vi "Verify with 3 Scrubbers.vi"(8 "error in":errorcluster) -> (0 "error out":errorcluster)   [LabVIEW 2020, in "Scrubber.Tests.lvclass"]
uses:
  Scrubber.Tests.lvclass
  Source/Approval Tests/Options/Options.lvclass
  Source/Approval Tests/Regex Scrubber/Regex Scrubber.lvclass
  C:/Users/SAS/Desktop/ApprovalTests.LabVIEW/Source/Approval Tests/Scrubber/Scrubber.lvclass
  Source/Approval Tests/Regex Scrubber/Regex Scrubber.lvclass/Regex Scrubber.ctl
  Source/Approval Tests/Options/Options.lvclass/Options.ctl
  Source/Approval Tests/Naming Data/Naming Data.lvclass/Naming Data.ctl
  4b862e9e-fcb2-487f-ab73-d9f83fbf4d2c.vi
  Source/Approval Tests/Regex Scrubber/Write Regex.vi
  Source/Approval Tests/Regex Scrubber/Write Replacement.vi
  4b862e9e-fcb2-487f-ab73-d9f83fbf4d2c.vi/500b534b-d6f0-4fa5-90b2-c40158375321.vi
  Source/Approval Tests/Update Test Name if Not Defined.vi
  4b862e9e-fcb2-487f-ab73-d9f83fbf4d2c.vi/500b534b-d6f0-4fa5-90b2-c40158375321.vi/93c5622b-9fb7-41e0-8c76-3fde37e94e34.vi
  Source/Approval Tests/Verify Core.vi
  Source/Approval Tests/Options/Read Scrubber.vi
  Source/Approval Tests/Naming Data/Read Test VI Name.vi
  Source/Approval Tests/Naming Data/Write Test VI Name.vi
  4b862e9e-fcb2-487f-ab73-d9f83fbf4d2c.vi/500b534b-d6f0-4fa5-90b2-c40158375321.vi/93c5622b-9fb7-41e0-8c76-3fde37e94e34.vi/04cb982b-2eda-40d0-8d7e-90f8e0b569b2.vi
  Source/Approval Tests/Options/Read Namer.vi
  Source/Approval Tests/Options/Read Naming Data.vi
  Source/Approval Tests/Options/Read Reporter.vi
  Source/Approval Tests/Options/Write Add Scrubber.vi
  Source/Approval Tests/conv EOL.vi
  <vilib>/Utility/libraryn.llb/Check if File or Folder Exists.vi
  Source/Approval Tests/Reporter/Report.vi
  <vilib>/addons/_JKI Toolkits/Caraya/classes/Assert/Assert.vi
  <vilib>/addons/_JKI Toolkits/Caraya/classes/Assert/Assert True.vi
  Source/Approval Tests/Scrubber/Scrubber.lvclass
  Source/Approval Tests/Namer/Namer.lvclass
  Source/Approval Tests/Naming Data/Naming Data.lvclass
  Source/Approval Tests/Reporter/Reporter.lvclass
  Scrubber.Tests.lvclass/Scrubber.Tests.ctl
  <vilib>/addons/_JKI Toolkits/Caraya/classes/Test/Test.lvclass
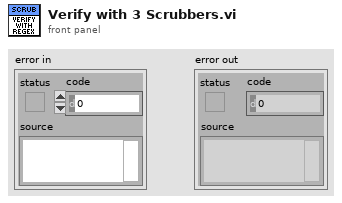
[diagram p1: front panel]
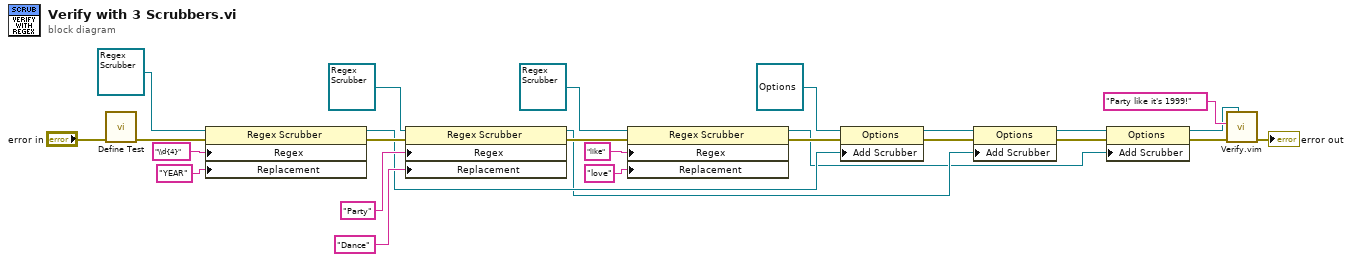
[diagram p0: block diagram]
diagram:
  n1 = call <vilib>:"Define Test.vi"("error in (no error)"="error in") -> ("error out"=w26:errorcluster)  [unwired: 9 in, 1 out]
  n2 = property class="Regex Scrubber"(reference=refnum<class "Regex Scrubber.lvclass"> refnum ("Approval Tests.lvlib:Regex Scrubber.lvclass"), error in=w26, "Regex"="\\d{4}", "Replacement"="YEAR") -> (reference out=w9:refnum<class "Regex Scrubber.lvclass">, error out=w23:errorcluster)
  n3 = property class="Regex Scrubber"(reference=refnum<class "Regex Scrubber.lvclass"> refnum ("Approval Tests.lvlib:Regex Scrubber.lvclass"), error in=w23, "Regex"="Party", "Replacement"="Dance") -> (reference out=w7:refnum<class "Regex Scrubber.lvclass">, error out=w22:errorcluster)
  n4 = property class="Regex Scrubber"(reference=refnum<class "Regex Scrubber.lvclass"> refnum ("Approval Tests.lvlib:Regex Scrubber.lvclass"), error in=w22, "Regex"="like", "Replacement"="love") -> (reference out=w1:refnum<class "Regex Scrubber.lvclass">, error out=w18:errorcluster)
  n5 = property class="Options"(reference=refnum<class "Options.lvclass"> refnum ("Approval Tests.lvlib:Options.lvclass"), error in=w18, "Add Scrubber"=w9) -> (reference out=w8:refnum<class "Options.lvclass">, error out=w21:errorcluster)
  n6 = property class="Options"(reference=w8, error in=w21, "Add Scrubber"=w7) -> (reference out=w6:refnum<class "Options.lvclass">, error out=w20:errorcluster)
  n7 = property class="Options"(reference=w6, error in=w20, "Add Scrubber"=w1) -> (reference out=w5:refnum<class "Options.lvclass">, error out=w19:errorcluster)
  n8 = call "Verify.vim"("Options"=w5, "error in"=w19, "Test Data"="Party like it's 1999!") -> ("error out"=→"error out":errorcluster)  [unwired: 7 in, 1 out]
